vi "Gaussian_Centered_4(SubVI).vi"(7 "Frequency (MHz)":dbl, 9 "Amplitude":dbl, 10 "Envelope Decay Time (micro s)":dbl, 11 "Number Of Points(integer multiple of 4096)":i32) -> ()   [LabVIEW 2016]
panel:
  out "output waveform 2":waveform(dbl)(graph)
  in  "High Voltage Width (us)":dbl
  in  "file path (use dialog)":path
  out "output waveform":waveform(dbl)(graph)
  in  "DAC frequency (MHz)":dbl
  # "Amplitude should not exceed 1.46V"
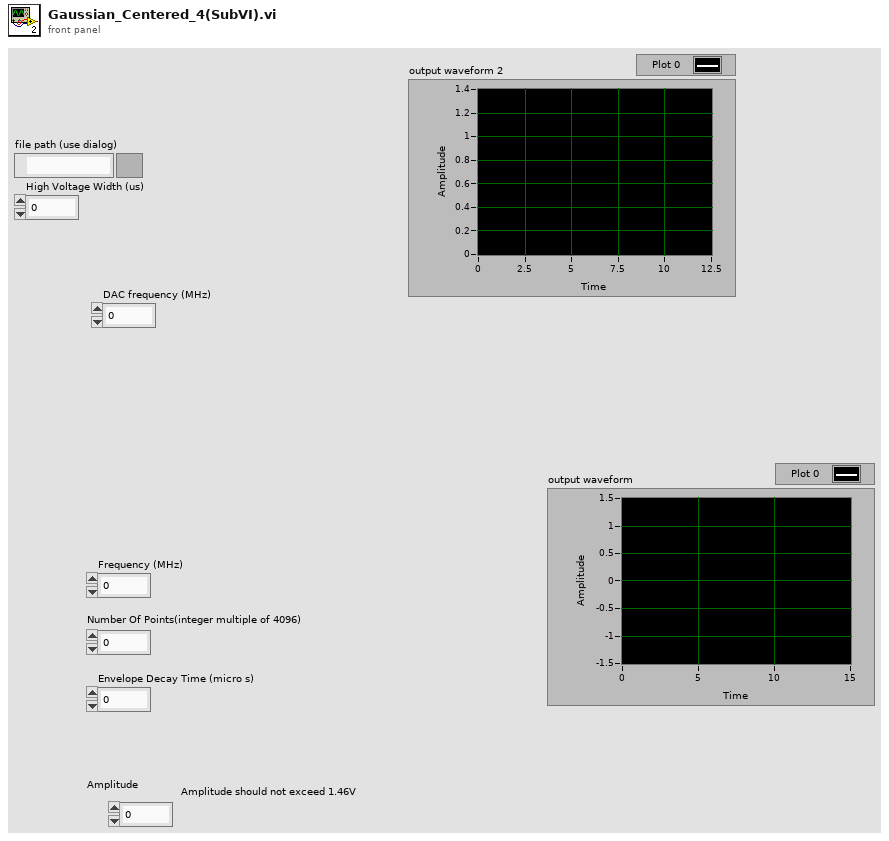
[diagram p1: front panel]
types:
  T1 = enum16{"open", "replace", "create", "open or create", "replace or create", "replace or create with confirmation"}
  T2 = enum16{"big-endian, network order", "native, host order", "little-endian"}
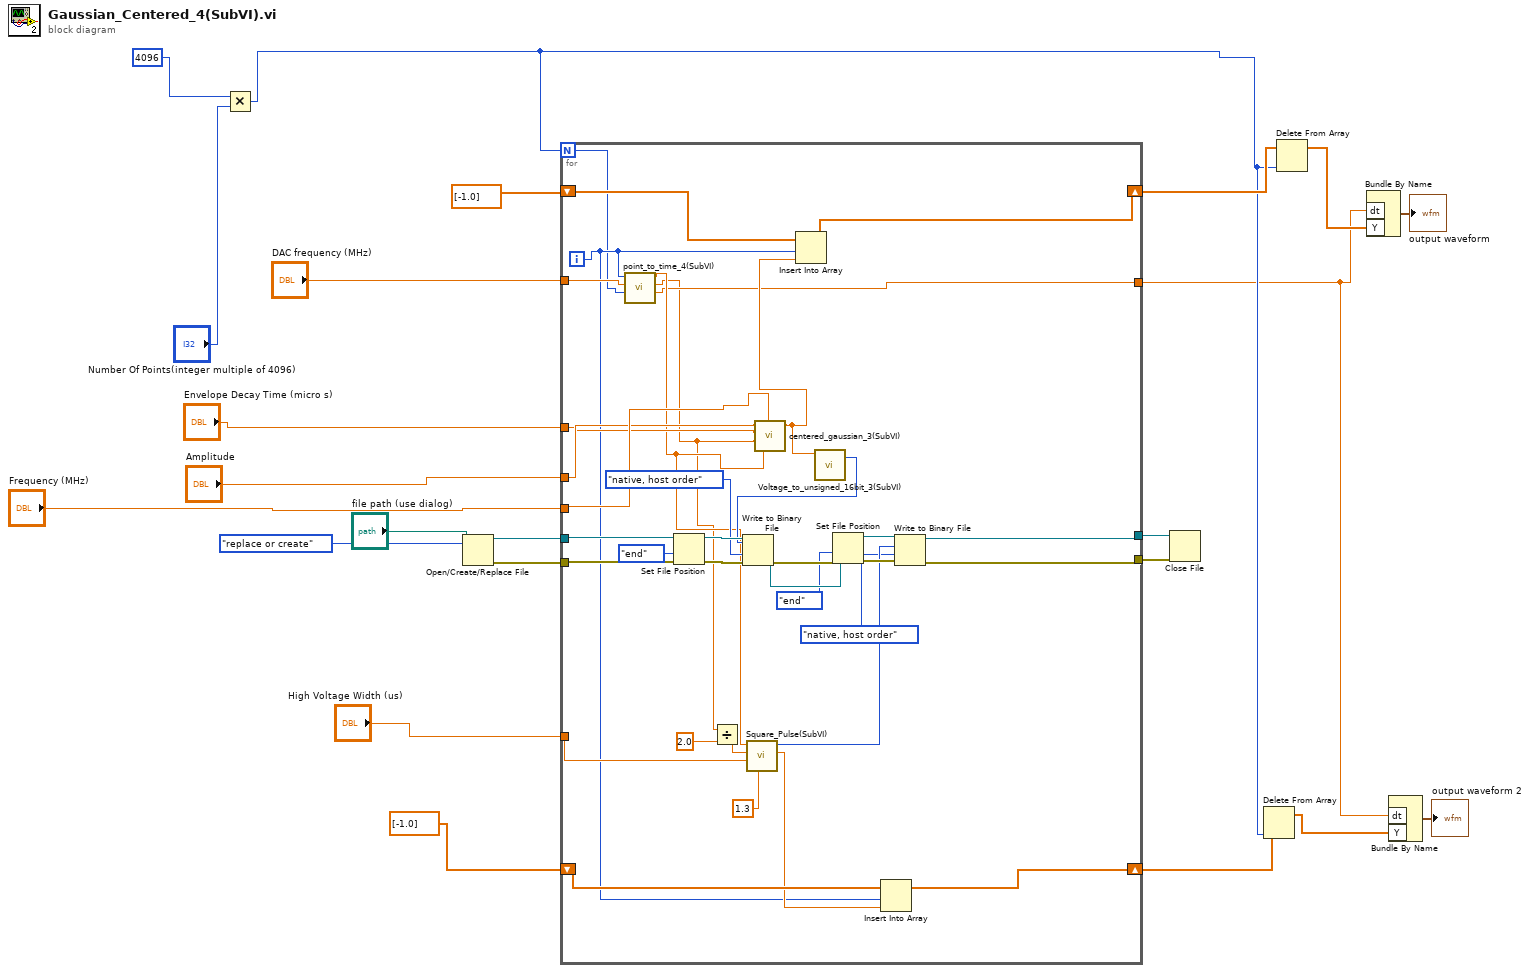
[diagram p0: block diagram]
diagram:
  n1 = Multiply(x=4096, y="Number Of Points(integer multiple of 4096)") -> (x*y=w5:i32)
  n2 = Open/Create/Replace File(file path (use dialog)="file path (use dialog)", operation (0:open)=T1."replace or create") -> (refnum out=w12:refnum<file>, error out=w11:errorcluster)  [unwired: 4 in, 1 out]
  n3 = for {
    N: w5 -> [w27]
    tunnel: "Amplitude" -> [w47]
    shift-right: [w57] -> w8
    shift-left: dbl[] [-1.0] ("array") -> [w58]
    tunnel: "Envelope Decay Time (micro s)" -> [w46]
    tunnel: "Frequency (MHz)" -> [w49]
    tunnel: "DAC frequency (MHz)" -> [w29]
    tunnel: [w25] -> w3
    tunnel: w12 -> [w56]
    tunnel: w11 -> [w55]
    tunnel: [w32] -> w10
    tunnel: [w31] -> w9
    tunnel: "High Voltage Width (us)" -> [w44]
    shift-right: [w41] -> w6
    shift-left: dbl[] [-1.0] ("array") -> [w43]
    i -> [w28]
    n4 = call "point_to_time_4(SubVI).vi"("number of points"=w27, "DAC frequency(MHz)"=w29, "point location"=w28) -> ("dt (us)"=w25:dbl, "Pulse Width (us)"=w24:dbl, "time (us)"=w26:dbl)  [unwired: 6 in]
    n5 = Set File Position(refnum=w56, from (0:start)=enum16{"start", "end", "current"}."end", error in=w55) -> (refnum out=w54:refnum<file>, error out=w53:errorcluster)  [unwired: 1 in]
    n6 = Divide(x=w24, y=2.0) -> (x/y=w40:dbl)
    n7 = call "Square_Pulse(SubVI).vi"("High Voltage (V)"=1.3, "High Voltage Width (us)"=w44, "Pulse Center (us)"=w40, "Time"=w26) -> ("Voltage Out"=w42:dbl, "unsigned 16-bit out"=w33:u16)  [unwired: 6 in]
    n8 = call "centered_gaussian_3(SubVI).vi"("time"=w26, "Frequency(MHz)"=w49, "Pulse Spacing"=w24, "Envelope DecayTime(micro s)"=w46, "Amplitude"=w47) -> ("output"=w48:dbl)  [unwired: 6 in]
    n9 = Insert Into Array(array=w58, index=w28, new element=w48) -> (w57:dbl[])
    n10 = call "Voltage_to_unsigned_16bit_3(SubVI).vi"("Voltage_in"=w48) -> ("unsigned 16bit integer"=w50:u16)  [unwired: 10 in]
    n11 = Write to Binary File(file (use dialog)=w54, data=w50, error in=w53, 9:T2."native, host order" ("byte order (0:big-endian, network order)")) -> (refnum out=w38:refnum<file>, error out=w37:errorcluster)  [unwired: 2 in, 1 out]
    n12 = Set File Position(refnum=w38, from (0:start)=enum16{"start", "end", "current"}."end", error in=w37) -> (refnum out=w35:refnum<file>, error out=w34:errorcluster)  [unwired: 1 in]
    n13 = Insert Into Array(array=w43, index=w28, new element=w42) -> (w41:dbl[])
    n14 = Write to Binary File(file (use dialog)=w35, data=w33, error in=w34, 9:T2."native, host order" ("byte order (0:big-endian, network order)")) -> (refnum out=w32:refnum<file>, error out=w31:errorcluster)  [unwired: 2 in, 1 out]
  }
  n15 = Close File(refnum=w10, error in=w9) -> ()  [unwired: 2 out]
  n16 = Delete From Array(array=w6, index=w5) -> (array with subset deleted=w4:dbl[])  [unwired: 1 in, 1 out]
  n17 = Delete From Array(array=w8, index=w5) -> (array with subset deleted=w15:dbl[])  [unwired: 1 in, 1 out]
  n18 = Bundle By Name("dt"=w3, "Y"=w15) -> (→"output waveform":waveform(dbl))  [unwired: 1 in]
  n19 = Bundle By Name("dt"=w3, "Y"=w4) -> (→"output waveform 2":waveform(dbl))  [unwired: 1 in]
